vi "test_Bitfile Reload_DMA Data Type Change.vi"(8 "error in (no error)":errorcluster, 11 "TestCase in":refnum<class "FPGA Addon Bitfile Reload Unit Tests.lvclass">) -> (0 "error out":errorcluster, 3 "TestCase out":refnum<class "FPGA Addon Bitfile Reload Unit Tests.lvclass">)   [LabVIEW 2021, in "FPGA Addon Bitfile Reload Unit Tests.lvclass"]
uses:
  FPGA Addon Bitfile Reload Unit Tests.lvclass
  Addon/Addon Shared/Types/DMA Information.ctl
  Addon/Addon Shared/Types/FPGA Addon Data Type.ctl
  Addon/Addon Shared/Types/DMA Settings.ctl
  Addon/Addon Shared/Types/Delacing Scheme.ctl
  Addon/Addon Shared/Types/DMA Acquisition Mode.ctl
  <vilib>/addons/_JKI Toolkits/VI Tester/TestCase.llb/TestCase.lvclass
  Addon/Addon Shared/FPGA Addon Shared.lvlib
  FPGA Addon Test Class/FPGA Addon Test Class.lvclass
  APIs/Scripting API/Scripting API.lvlib
  Addon/Addon System Explorer/FPGA Addon System Explorer.lvlib
  C:/Program Files/National Instruments/LabVIEW 2021/vi.lib/addons/_JKI Toolkits/VI Tester/TestCase.llb/TestCase.lvclass
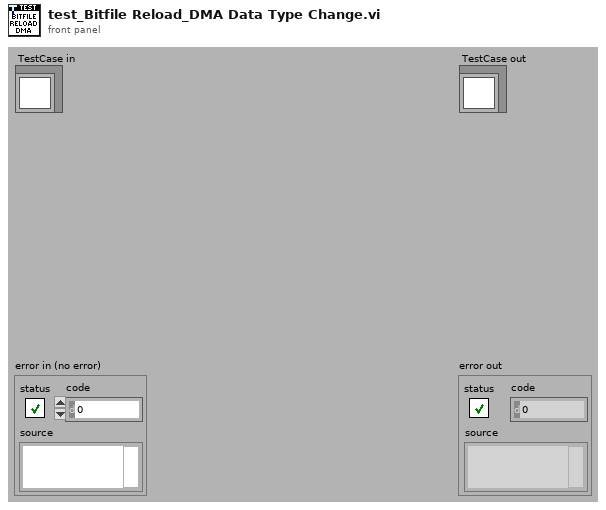
[diagram p1: front panel]
types:
  T1 = typedef "FPGA Addon Shared.lvlib/DMA Settings.ctl" = cluster{"Number of Channels":u8, "Delacing Scheme":T2, "Update Rate":u32, "dt":dbl, "Mode":T3, "Number of Samples":u32, "DMA Host Buffer":u32}
  T2 = typedef "FPGA Addon Shared.lvlib/Delacing Scheme.ctl" = enum8{"Interleaved", "Bitpacked"}
  T3 = typedef "FPGA Addon Shared.lvlib/DMA Acquisition Mode.ctl" = enum8{"Continuous", "Triggered Finite"}
  T4 = typedef "FPGA Addon Shared.lvlib/DMA Information.ctl" = cluster{"Name":string, "Data Type":T5}
  T5 = typedef "FPGA Addon Shared.lvlib/FPGA Addon Data Type.ctl" = enum8{"<Null>", "I8", "I16", "I32", "I64", "U8", "U16", "U32", "U64", "SGL", "Boolean", "Analog PWM In Settings", "Analog PWM In", "Digital PWM In Settings", "Digital PWM In", "Digital PWM Out", "Sine Out", "FXP", "FXP+/-24.5", "FXP+/-16.5", "FXP+/-32.8", "FXP+/-64.32", "FXP+/-16.7", "FXP+/-20.5", "FXP+/-27.5", "FXP+/-32.16", "FXP+16.3", "FXP+18.3", "Digital Static In", "Digital Static Out", "Digital Static In Settings", "Digital WSS Out", "Quad Encoder Settings", "Quad Encoder In", "Group"}
  T6 = typedef "Custom Device API.lvlib/Custom Device Item Ref.ctl" = u64
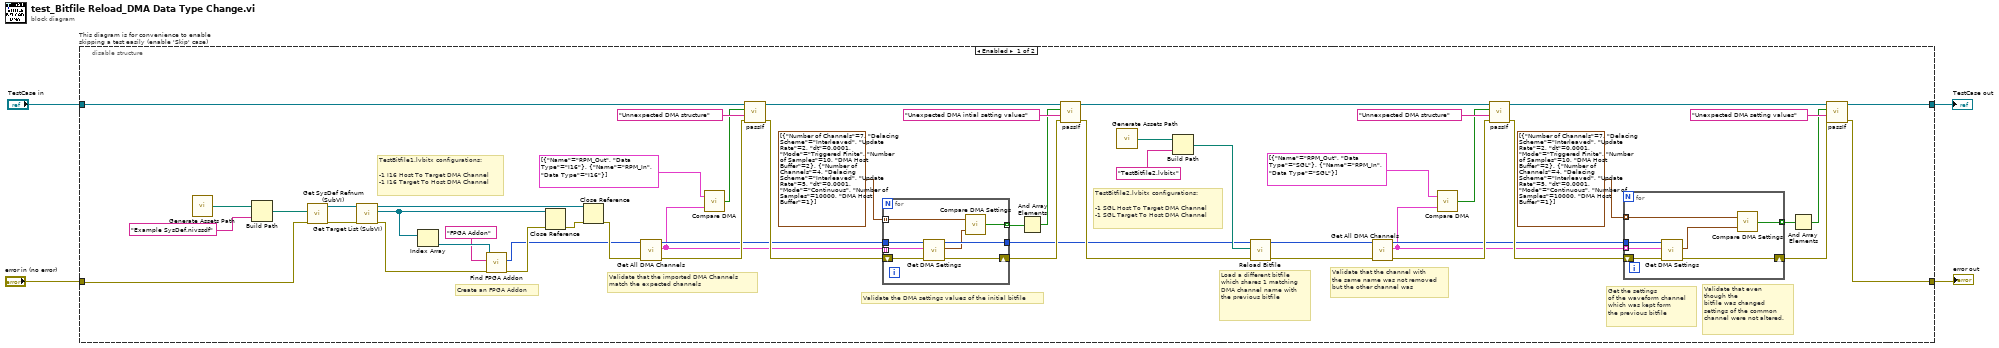
[diagram p0: block diagram]
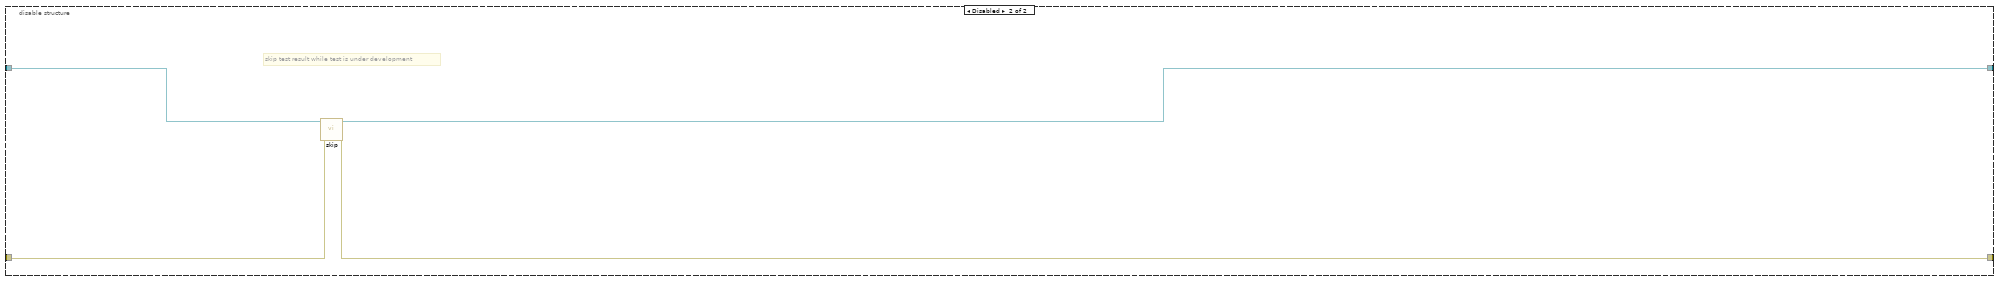
[diagram p2: hidden frame]
diagram:
  n1 = disable-structure "This diagram is for convenience to enable skipping a test easily (enable 'Skip' case)" shown="Enabled" {
    disable-tunnel: "TestCase in" -> [w31 w75]
    disable-tunnel: [w22 w73] -> w1
    disable-tunnel: [w23 w74] -> w3
    disable-tunnel: "error in (no error)" -> [w30 w72]
    frame Enabled {
      # "TestBitfile1.lvbitx configurations:\n\n-1 I16 Host To Target DMA Channel\n-1 I16 Target To Host DMA Channel"
      # "Validate the DMA settings values of the initial bitfile"
      # "Validate that even \nthough the \nbitfile was changed\nsettings of the common \nchannel were not altered."
      # "Get the settings \nof the waveform channel\nwhich was kept form \nthe previous bitfile"
      # "TestBitfile2.lvbitx configurations:\n\n-1 SGL Host To Target DMA Channel\n-1 SGL Target To Host DMA Channel"
      # "Validate that the channel with \nthe same name was not removed\nbut the other channel was"
      # "Load a different bitfile\nwhich shares 1 matching\nDMA channel name with \nthe previous bitfile"
      # "Validate that the imported DMA Channels \nmatch the expected channels"
      # "Create an FPGA Addon"
      n2 = call "Generate Assets Path.vi"() -> ("Assets path"=w48:path)
      n3 = Build Path(base path=w48, name or relative path="Example SysDef.nivssdf") -> (appended path=w55:path)
      n4 = call "Get SysDef Refnum (SubVI).vi"("error in (no error)"=w30, "System Definition path"=w55) -> ("error out"=w53:errorcluster, "SysDef Refnum out"=w54:refnum<k24>)  [unwired: 8 in]
      n5 = call "Get Target List (SubVI).vi"("error in (no error)"=w53, "SysDef Refnum in"=w54) -> ("error out"=w43:errorcluster, "Target List Refnums"=w52:refnum<k24>[], "SysDef Refnum out"=w51:refnum<k24>)  [unwired: 7 in]
      n6 = Index Array(array=w52) -> (element=w41:refnum<k24>)  [unwired: 1 in]
      n7 = call "Find FPGA Addon.vi"("error in"=w43, "FPGA addon name"="FPGA Addon", "target in"=w41) -> ("error out"=w42:errorcluster, "FPGA addon refnum out"=w38:T6)  [unwired: 5 in, 2 out]
      n8 = Close Reference(reference=w52, error in (no error)=w42) -> (error out=w50:errorcluster)
      n9 = Close Reference(reference=w51, error in (no error)=w50) -> (error out=w39:errorcluster)
      n10 = call "Get All DMA Channels.vi"("error in (no error)"=w39, "FPGA addon refnum in"=w38) -> ("error out"=w37:errorcluster, "DMA channels out"=w12:T4[], "FPGA addon refnum out"=w15:T6)  [unwired: 7 in]
      n11 = call "Compare DMA.vi"("Target bitfile DMA in"=w12, "Reference bitfile DMA in"=T4[] [{"Name"="RPM_Out", "Data Type"=enum."I16"}, {"Name"="RPM_In", "Data Type"=enum."I16"}] ("DMA channels out")) -> ("Equal ?"=w36:bool)
      n12 = call-dynamic "passIf.vi"("error in (no error)"=w37, "message (\"\")"="Unnexpected DMA structure" ("message (\"\")"), "pass"=w36, "TestCase in"=w31) -> ("error out"=w19:errorcluster, "TestCase out"=w21:refnum<class "FPGA Addon Bitfile Reload Unit Tests.lvclass">)  [unwired: 6 in]
      n13 = for {
        tunnel: w15 -> [w69]
        tunnel: [w68] -> w14
        shift-right: [w70] -> w17
        shift-left: w19 -> [w71]
        tunnel: w12 -> [w67] mode=indexing
        tunnel: T1[] [{"Number of Channels"=7, "Delacing Scheme"=enum."Interleaved", "Update Rate"=2, "dt"=0.0001, "Mode"=enum."Triggered Finite", "Number of Samples"=10, "DMA Host Buffer"=2}, {"Number of Channels"=4, "Delacing Scheme"=enum."Interleaved", "Update Rate"=5, "dt"=0.0001, "Mode"=enum."Continuous", "Number of Samples"=10000, "DMA Host Buffer"=1}] ("Array") -> [w65] mode=indexing
        tunnel: [w64] -> w10 mode=indexing
        n14 = call "Get DMA Settings.vi"("error in (no error)"=w71, "DMA Channel in"=w67, "FPGA addon refnum in"=w69) -> ("error out"=w70:errorcluster, "DMA Settings"=w66:T1, "FPGA addon refnum out"=w68:T6)  [unwired: 6 in]
        n15 = call "Compare DMA Settings.vi"("DMA Settings 2"=w66, "DMA Settings 1"=w65) -> ("equal?"=w64:bool)
      }
      n16 = And Array Elements(Boolean array=w10) -> (logical AND=w9:bool)
      n17 = call-dynamic "passIf.vi"("error in (no error)"=w17, "message (\"\")"="Unexpected DMA intial setting values" ("message (\"\")"), "pass"=w9, "TestCase in"=w21) -> ("error out"=w16:errorcluster, "TestCase out"=w20:refnum<class "FPGA Addon Bitfile Reload Unit Tests.lvclass">)  [unwired: 6 in]
      n18 = call "Generate Assets Path.vi"() -> ("Assets path"=w46:path)
      n19 = Build Path(base path=w46, name or relative path="TestBitfile2.lvbitx") -> (appended path=w45:path)
      n20 = call "Reload Bitfile.vi"("error in (no error)"=w16, "NewVal"=w45, "Item Ref in"=w14) -> ("error out"=w35:errorcluster, "Section Ref out"=w33:T6)  [unwired: 7 in]
      n21 = call "Get All DMA Channels.vi"("error in (no error)"=w35, "FPGA addon refnum in"=w33) -> ("error out"=w34:errorcluster, "DMA channels out"=w8:T4[], "FPGA addon refnum out"=w25:T6)  [unwired: 7 in]
      n22 = call "Compare DMA.vi"("Target bitfile DMA in"=w8, "Reference bitfile DMA in"=T4[] [{"Name"="RPM_Out", "Data Type"=enum."SGL"}, {"Name"="RPM_In", "Data Type"=enum."SGL"}] ("DMA channels out")) -> ("Equal ?"=w32:bool)
      n23 = call-dynamic "passIf.vi"("error in (no error)"=w34, "message (\"\")"="Unnexpected DMA structure" ("message (\"\")"), "pass"=w32, "TestCase in"=w20) -> ("error out"=w27:errorcluster, "TestCase out"=w28:refnum<class "FPGA Addon Bitfile Reload Unit Tests.lvclass">)  [unwired: 6 in]
      n24 = for {
        tunnel: w25 -> [w61]
        shift-right: [w62] -> w26
        shift-left: w27 -> [w63]
        tunnel: w8 -> [w60] mode=indexing
        tunnel: T1[] [{"Number of Channels"=7, "Delacing Scheme"=enum."Interleaved", "Update Rate"=2, "dt"=0.0001, "Mode"=enum."Triggered Finite", "Number of Samples"=10, "DMA Host Buffer"=2}, {"Number of Channels"=4, "Delacing Scheme"=enum."Interleaved", "Update Rate"=5, "dt"=0.0001, "Mode"=enum."Continuous", "Number of Samples"=10000, "DMA Host Buffer"=1}] ("Array") -> [w58] mode=indexing
        tunnel: [w57] -> w6 mode=indexing
        n25 = call "Get DMA Settings.vi"("error in (no error)"=w63, "DMA Channel in"=w60, "FPGA addon refnum in"=w61) -> ("error out"=w62:errorcluster, "DMA Settings"=w59:T1)  [unwired: 6 in, 1 out]
        n26 = call "Compare DMA Settings.vi"("DMA Settings 2"=w59, "DMA Settings 1"=w58) -> ("equal?"=w57:bool)
      }
      n27 = And Array Elements(Boolean array=w6) -> (logical AND=w5:bool)
      n28 = call-dynamic "passIf.vi"("error in (no error)"=w26, "message (\"\")"="Unexpected DMA setting values" ("message (\"\")"), "pass"=w5, "TestCase in"=w28) -> ("error out"=w23:errorcluster, "TestCase out"=w22:refnum<class "FPGA Addon Bitfile Reload Unit Tests.lvclass">)  [unwired: 6 in]
    }
    frame Disabled {
      # "skip test result while test is under development"
      n29 = call <vilib>:"skip.vi"("error in (no error)"=w72, "TestCase in"=w75) -> ("error out"=w74:errorcluster, "TestCase out"=w73:refnum<class "FPGA Addon Bitfile Reload Unit Tests.lvclass">)  [unwired: 8 in]
    }
  }
  "error out" <- w3
  "TestCase out" <- w1
